vi "Test_WriteItem_ClearTable_ReadItem_NoneReturned.vi"(8 "error in (no error)":errorcluster, 11 "TestCase in":refnum<class "TestComposedLookupTable.lvclass">) -> (0 "error out":errorcluster, 3 "TestCase out":refnum<class "TestComposedLookupTable.lvclass">)   [LabVIEW 2017, in "TestComposedLookupTable.lvclass"]
uses:
  TestComposedLookupTable.lvclass
  Source/LookupTable/LookupTable.lvclass/LookupTable.ctl
  87404576-7c1b-47e7-8bc2-e5fc3b6d3934.vi
  67c07c66-17b5-4699-8177-663ff06f665c.vi
  Source/LookupTable/Read Table Reference.vi
  87404576-7c1b-47e7-8bc2-e5fc3b6d3934.vi/1bfbdad6-7fe4-4a60-a547-4af39c3ee767.vi
  67c07c66-17b5-4699-8177-663ff06f665c.vi/82a74bc2-079c-4fce-88c6-43d70c30e506.vi
  Source/LookupTable/LookupTable.lvclass
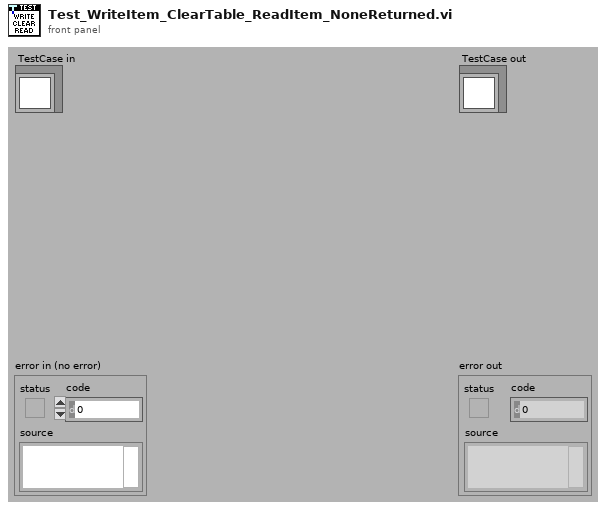
[diagram p1: front panel]
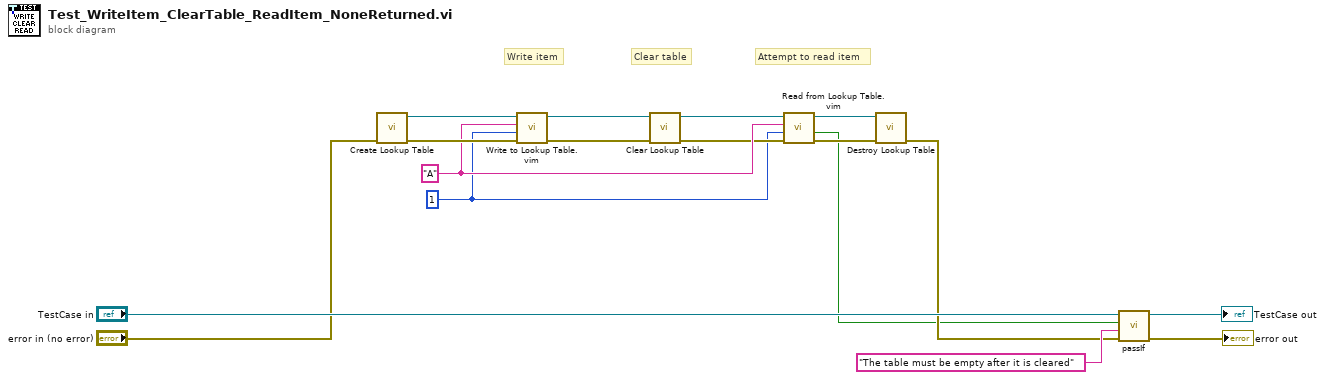
[diagram p0: block diagram]
diagram:
  w2 = 1
  w12 = "A" ("Item Name")
  # "Attempt to read item"
  # "Clear table"
  # "Write item"
  n1 = call "Create Lookup Table.vi"("error in (no error)"="error in (no error)") -> ("error out"=w17:errorcluster, "LookupTable Reference"=w7:refnum<data-value>)  [unwired: 9 in]
  n2 = call "Write to Lookup Table.vim"("error in (no error)"=w17, "Item"=w2, "Item Name"=w12, "LookupTable Reference"=w7) -> ("error out"=w9:errorcluster, "LookupTable Reference Out"=w4:refnum<data-value>)  [unwired: 5 in, 1 out]
  n3 = call "Clear Lookup Table.vi"("error in (no error)"=w9, "LookupTable Reference"=w4) -> ("error out"=w5:errorcluster, "LookupTable Reference Out"=w3:refnum<data-value>)  [unwired: 8 in]
  n4 = call "Read from Lookup Table.vim"("error in (no error)"=w5, "Type"=w2, "Item Name"=w12, "LookupTable Reference"=w3) -> ("error out"=w6:errorcluster, "Not Found?"=w1:bool, "LookupTable Reference Out"=w10:refnum<data-value>)  [unwired: 4 in, 1 out]
  n5 = call "Destroy Lookup Table.vi"("error in (no error)"=w6, "LookupTable Reference"=w10) -> ("error out"=w8:errorcluster)  [unwired: 9 in]
  n6 = call-dynamic "passIf.vi"("error in (no error)"=w8, "message (\"\")"="The table must be empty after it is cleared" ("message (\"\")"), "pass"=w1, "TestCase in"="TestCase in") -> ("error out"=→"error out":errorcluster, "TestCase out"=→"TestCase out":refnum<class "TestComposedLookupTable.lvclass">)  [unwired: 6 in]
